vi "AssertAllItems.vi"(0 "VI Reference In":refnum<vi>, 1 "Test Label":string, 2 "delimiter (>>)":string=">>", 3 "Assert Only? (F)":bool, 5 "Control Path":string, 7 "Item Names":string[](array[string]), 11 "Error In":errorcluster, 12 "Assert Interval(10 ms)":u32=10, 13 "Timeout(5 sec)":dbl=5.0) -> (4 "VI Reference Out":refnum<vi>, 6 "Asserted Value":string[](array[string]), 15 "Error Out":errorcluster)   [LabVIEW 2016, in "Drona.lvlib" / "AssertControlValue.lvlib" / "AssertListbox.lvlib"]
doc: "Asserts if all the items present in the listbox control is equal.\n\nThe input control name is given as a string , incase of path, use delimiters inbetween the path.\nThis VI gets the value of the control, untill the value is equal to the input value."
uses:
  AssertListbox.lvlib
  Get/GetControlRef/GetControlRefByPath.vi
  <vilib>/addons/_JKI Toolkits/Caraya/classes/Assert/Assert Equal Value_Variant.vi
  <vilib>/addons/_JKI Toolkits/Caraya/classes/Assert/Assert.lvclass
  Get/GetControlRef/GetControlRef.lvlib
panel:
  # "Need to confirm if we need to \nsort the item names before assert?"
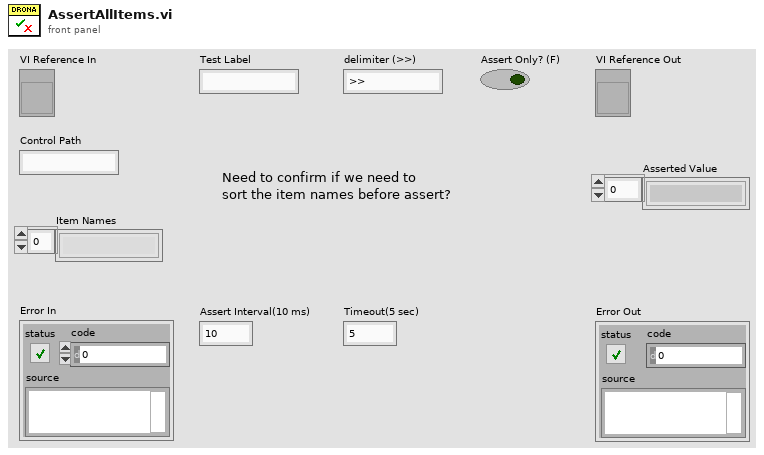
[diagram p1: front panel]
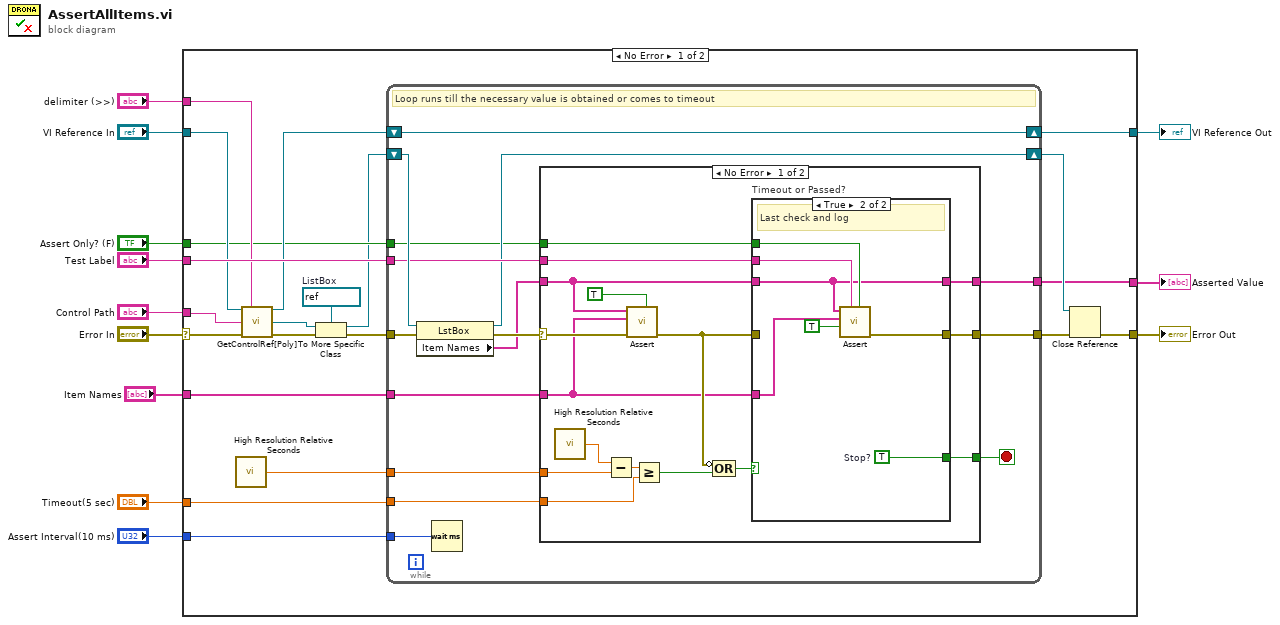
[diagram p0: block diagram]
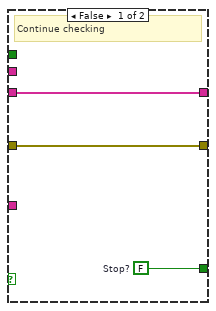
[diagram p2: hidden frame]
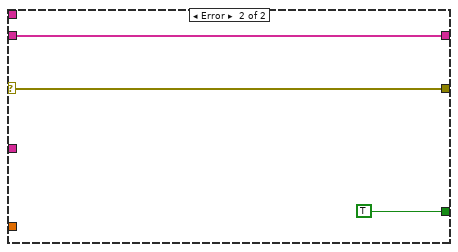
[diagram p3: hidden frame]
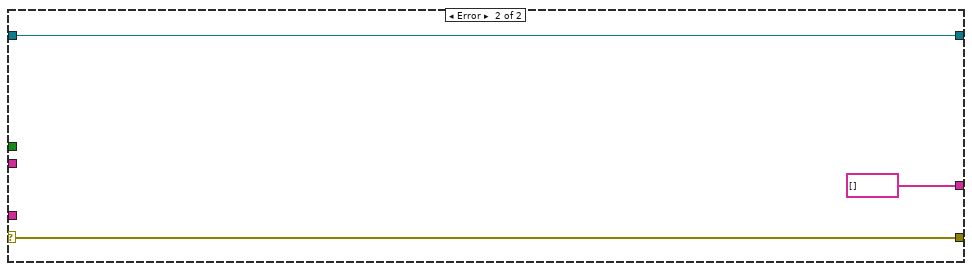
[diagram p4: hidden frame]
diagram:
  n1 = case shown="No Error" "Error In" {
    selector: "Error In" -> [w28 w80]
    tunnel: "Timeout(5 sec)" -> [w33 _]
    tunnel: [w32 w79] -> w11
    tunnel: [w22 w80] -> w10
    tunnel: "Assert Interval(10 ms)" -> [w30 _]
    tunnel: "Test Label" -> [w29 _]
    tunnel: "VI Reference In" -> [w27 w79]
    tunnel: "Control Path" -> [w26 _]
    tunnel: "delimiter (>>)" -> [w20 _]
    tunnel: "Assert Only? (F)" -> [w19 _]
    tunnel: [w18 string[] [] ("Item Names")] -> w1
    tunnel: "Item Names" -> [w13 _]
    frame No Error {
      w15 = refnum<vi> refnum  # ListBox
      n2 = call <vilib>:"High Resolution Relative Seconds.vi"() -> ("relative seconds"=w25:dbl)
      n3 = call-poly "GetControlRef[Poly].vi"("VI Reference In"=w27, "delimiter (>>)"=w20, "Control Path"=w26, "error In"=w28) -> ("VI Reference Out"=w23:refnum<vi>, "Ctl Refnum"=w16:refnum<vi>, "error out"=w24:errorcluster)  [unwired: 9 in]
      n4 = To More Specific Class(target class=w15, reference=w16, error in=w24) -> (specific class reference=w14:refnum<vi>, error out=w17:errorcluster)
      n5 = while {
        tunnel: w33 -> [w47]
        tunnel: w25 -> [w48]
        tunnel: w17 -> [w42]
        tunnel: [w45] -> w31
        tunnel: w30 -> [w43]
        tunnel: w29 -> [w39]
        shift-right: [w40] -> w32
        shift-left: w23 -> [w40]
        shift-right: [w38] -> w21
        shift-left: w14 -> [w41]
        tunnel: w19 -> [w37]
        tunnel: [w36] -> w18
        tunnel: w13 -> [w35]
        stop <- w46 stop-if-true
        # "Loop runs till the necessary value is obtained or comes to timeout"
        n6 = property on="Property Node" class="LstBox"(reference=w41, error in=w42) -> (reference out=w38:refnum<vi>, error out=w44:errorcluster, "Item Names"=w34:string[])
        n7 = Wait (ms)(milliseconds to wait=w43) -> ()  [unwired: 1 out]
        n8 = case shown="No Error" w44 {
          selector: w44 -> [w60 w77]
          tunnel: w48 -> [w64 _]
          tunnel: w47 -> [w61 _]
          tunnel: [w52 TRUE] -> w46
          tunnel: [w53 w77] -> w45
          tunnel: w34 -> [w54 w75]
          tunnel: w39 -> [w59 _]
          tunnel: w37 -> [w51 _]
          tunnel: [w50 w75] -> w36
          tunnel: w35 -> [w49 _]
          frame No Error {
            n9 = call <vilib>:"High Resolution Relative Seconds.vi"() -> ("relative seconds"=w63:dbl)
            n10 = Subtract(x=w63, y=w64) -> (x-y=w62:dbl)
            n11 = call-poly <vilib>:"Assert.vi"("Assert Only? (F)"=TRUE, "error in (no error)"=w60, "Y"=w49, "X"=w54) -> ("error out"=w57:errorcluster)  [unwired: 7 in]
            n12 = Greater Or Equal?(x=w62, y=w61) -> (x >= y?=w58:bool)
            n13 = Compound Arithmetic op=OR(invert w57, w58) -> (w56:bool)
            n14 = case "Timeout or Passed?" shown="True" w56 {
              tunnel: w57 -> [w67 _]
              tunnel: w49 -> [_ w73]
              tunnel: w54 -> [w65 w68]
              tunnel: w59 -> [_ w74]
              tunnel: [w67 w72] -> w53
              tunnel: [w66 w71] -> w52
              tunnel: w51 -> [_ w69]
              tunnel: [w65 w68] -> w50
              frame False {
                w66 = FALSE  # Stop?
                # "Continue checking"
              }
              frame True {
                w71 = TRUE  # Stop?
                # "Last check and log"
                n15 = call-poly <vilib>:"Assert.vi"("Assert Only? (F)"=w69, "Label"=w74, "Register with caller test (F)"=TRUE, "Y"=w73, "X"=w68) -> ("error out"=w72:errorcluster)  [unwired: 6 in]
              }
            }
          }
          frame Error {
          }
        }
      }
      n16 = Close Reference(reference=w21, error in (no error)=w31) -> (error out=w22:errorcluster)
    }
    frame Error {
    }
  }
  "Error Out" <- w10
  "VI Reference Out" <- w11
  "Asserted Value" <- w1
